vi "rbind.vi"(11 "data":dbl[][](array[numeric])) -> (3 "data (cbind)":dbl[][](array[numeric]))   [LabVIEW 2014]
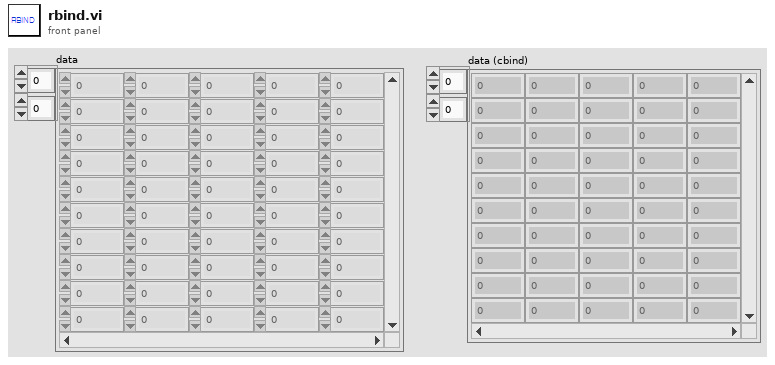
[diagram p1: front panel]
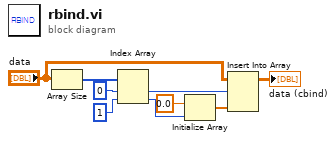
[diagram p0: block diagram]
diagram:
  n1 = Array Size(array="data") -> (size(s)=w3:i32[])
  n2 = Index Array(array=w3, index #1=0 ("index"), index #2=1 ("index")) -> (element #1=w1:i32, element #2=w6:i32)
  n3 = Initialize Array(0.0, w6) -> (w8:dbl[])
  n4 = Insert Into Array(array="data", index (row)=w1, new element=w8) -> (→"data (cbind)":dbl[][])  [unwired: 1 in]
